vi "close.vi"(8 "error in (no error)":errorcluster, 11 "midi-ui in":refnum<class "midi-ui.lvclass">) -> (0 "error out":errorcluster)   [LabVIEW 2020, in "midi-ui.lvclass"]
uses:
  midi-ui.lvclass
  midi-ui.lvclass/midi-ui.ctl
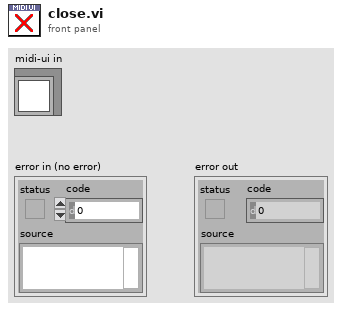
[diagram p1: front panel]
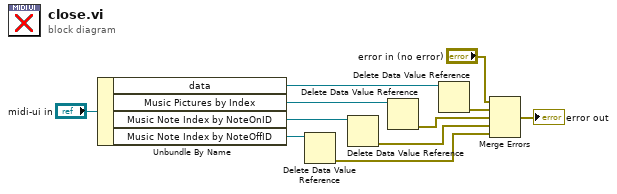
[diagram p0: block diagram]
diagram:
  n1 = Unbundle By Name("midi-ui in") -> ("data"=w10:refnum<data-value>, "Music Pictures by Index"=w4:refnum<data-value>, "Music Note Index by NoteOnID"=w5:refnum<data-value>, "Music Note Index by NoteOffID"=w6:refnum<data-value>)
  n2 = Delete Data Value Reference(data value reference=w6) -> (error out=w1:errorcluster)  [unwired: 1 in, 1 out]
  n3 = Delete Data Value Reference(data value reference=w5) -> (error out=w2:errorcluster)  [unwired: 1 in, 1 out]
  n4 = Delete Data Value Reference(data value reference=w4) -> (error out=w3:errorcluster)  [unwired: 1 in, 1 out]
  n5 = Delete Data Value Reference(data value reference=w10) -> (error out=w7:errorcluster)  [unwired: 1 in, 1 out]
  n6 = Merge Errors("error in (no error)", w7, w3, w2, w1) -> (→"error out":errorcluster)
